vi "DC calculator.vi"(11 "Subset 3":dbl[](array[numeric])) -> (3 "Numeric":dbl)   [LabVIEW 2018]
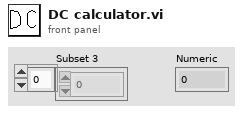
[diagram p1: front panel]
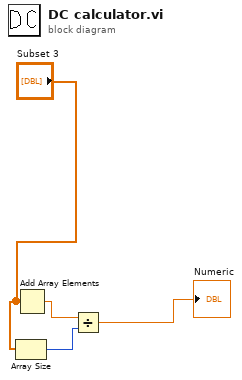
[diagram p0: block diagram]
diagram:
  n1 = Array Size(array="Subset 3") -> (size(s)=w3:i32)
  n2 = Add Array Elements(numeric array="Subset 3") -> (sum=w2:dbl)
  n3 = Divide(x=w2, y=w3) -> (x/y=→"Numeric":dbl)
